vi "TestApproachingZero.vi"() -> ()   [LabVIEW 2020]
doc: "Test program for Edge On"
panel:
  in  "Value":dbl
  out "count":i32
  out "ApproachingZero?":bool
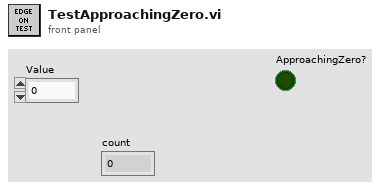
[diagram p1: front panel]
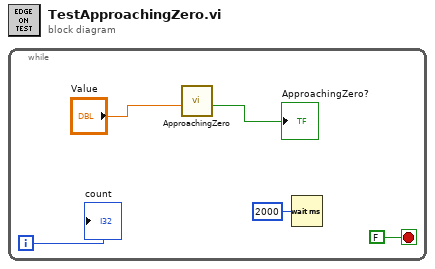
[diagram p0: block diagram]
diagram:
  n1 = while {
    i -> [w3]
    stop <- FALSE stop-if-true
    n2 = call "ApproachingZero.vi"("Value"="Value") -> ("IsAproachingZero?"=→"ApproachingZero?":bool)  [unwired: 10 in]
    n3 = Wait (ms)(milliseconds to wait=u32 2000) -> ()  [unwired: 1 out]
    "count" <- w3
  }
